vi "TMCM351- setActualPosition.vi"(4 "错误输入":errorcluster caption="错误输入（无错误）", 5 "Position":i32, 6 "motor":u8(ring) items=["x", "y", "z"], 7 "com in":refnum<visa-resource-name>) -> (0 "错误输出":errorcluster, 3 "com out":refnum<visa-resource-name>)   [LabVIEW 2018]
uses:
  module_param.vi
panel:
  # "设置分辨率"
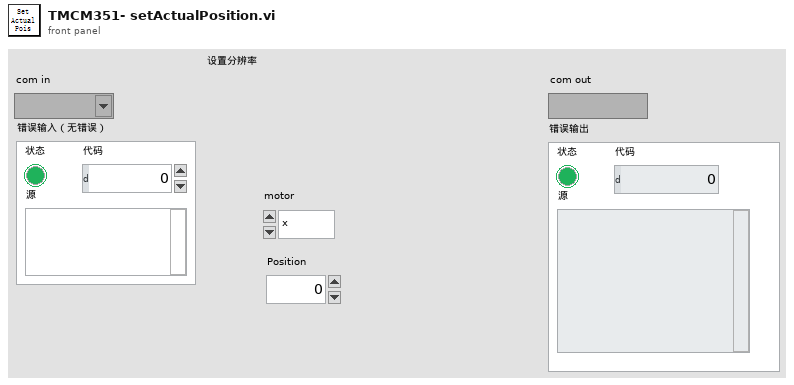
[diagram p1: front panel]
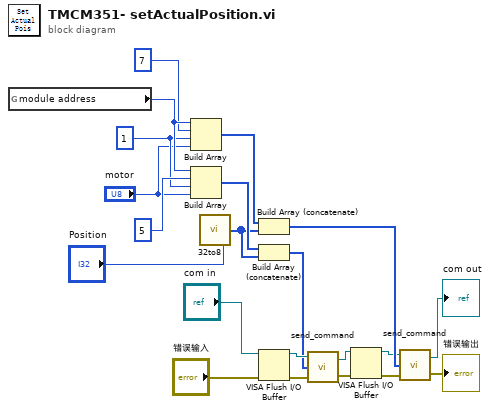
[diagram p0: block diagram]
diagram:
  w12 = u8 1
  n1 = global read "module_param.vi" "module address"() -> (w14:u8)
  n2 = Build Array(w14, u8 7 ("元素"), w12, "motor") -> (w10:u8[])
  n3 = Build Array(w14, u8 5, w12, "motor") -> (w16:u8[])
  n4 = call "32to8.vi"("32data_in"="Position") -> ("8Array"=w9:u8[])
  n5 = Build Array (concatenate)(w10, w9) -> (w8:u8[])
  n6 = Build Array (concatenate)(w16, w9) -> (w15:u8[])
  n7 = VISA Flush I/O Buffer(VISA resource name="com in", error in (no error)="错误输入") -> (VISA resource name out=w18:refnum<visa-resource-name>, error out=w17:errorcluster)  [unwired: 1 in]
  n8 = call "send_command.vi"("错误输入"=w17, 3:w15, "com in"=w18) -> ("错误输出"=w6:errorcluster, "com out"=w7:refnum<visa-resource-name>)
  n9 = VISA Flush I/O Buffer(VISA resource name=w7, error in (no error)=w6) -> (VISA resource name out=w5:refnum<visa-resource-name>, error out=w4:errorcluster)  [unwired: 1 in]
  n10 = call "send_command.vi"("错误输入"=w4, 3:w8, "com in"=w5) -> ("错误输出"=→"错误输出":errorcluster, "com out"=→"com out":refnum<visa-resource-name>)
